vi "Check Chain Types.vi"(8 "error in (no error)":errorcluster, 10 "Then":refnum<class "Promise.lvclass">, 11 "Future in":refnum<class "Future.lvclass">) -> (0 "error out":errorcluster, 3 "Future out":refnum<class "Future.lvclass">)   [LabVIEW 2020, in "Promises.lvlib" / "Future.lvclass"]
uses:
  Future.lvclass
  Future.lvclass/Future.ctl
  Promise/Promise.lvclass
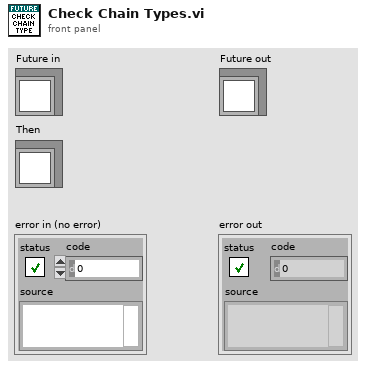
[diagram p1: front panel]
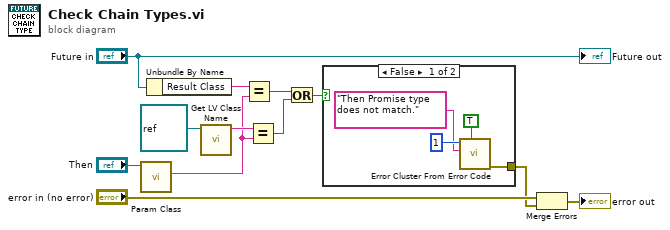
[diagram p0: block diagram]
diagram:
  n1 = call "Param Class.vi"("Promise in"="Then") -> ("Param Class"=w3:string)  [unwired: 10 in]
  n2 = Unbundle By Name("Future in") -> ("Result Class"=w10:string)
  n3 = call <vilib>:"Get LV Class Name.vi"("object"=refnum<class> refnum ("LabVIEW Object")) -> ("class name"=w4:string)  [unwired: 9 in, 1 out]
  n4 = Equal?(x=w10, y=w3) -> (x = y?=w9:bool)
  n5 = Equal?(x=w4, y=w3) -> (x = y?=w2:bool)
  n6 = Or(x=w9, y=w2) -> (x .or. y?=w6:bool)
  n7 = case shown="False" w6 {
    tunnel: [w16 _] -> w7
    frame False {
      n8 = call <vilib>:"Error Cluster From Error Code.vi"("show call chain? (False)"=TRUE, "error message (\"\")"="Then Promise type does not match." ("String In"), "error code (0)"=1) -> ("error out"=w16:errorcluster)  [unwired: 6 in]
    }
    frame True {
    }
  }
  n9 = Merge Errors("error in (no error)", w7) -> (→"error out":errorcluster)
  "Future out" <- "Future in"
